vi "contract inside.vi"(10 "xmax":dbl[](array[numeric]), 11 "centroid":dbl[](array[numeric])) -> (3 "xc":dbl[](array[numeric]))   [LabVIEW 2015]
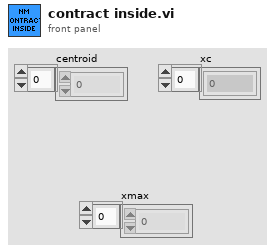
[diagram p1: front panel]
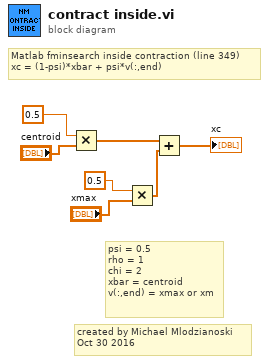
[diagram p0: block diagram]
diagram:
  # "Matlab fminsearch inside contraction (line 349)\nxc = (1-psi)*xbar + psi*v(:,end)"
  # "created by Michael Mlodzianoski\nOct 30 2016"
  # "psi = 0.5\nrho = 1\nchi = 2\nxbar = centroid\nv(:,end) = xmax or xm"
  n1 = Multiply(x=0.5, y="centroid") -> (x*y=w3:dbl[])
  n2 = Multiply(x=0.5, y="xmax") -> (x*y=w2:dbl[])
  n3 = Add(x=w3, y=w2) -> (x+y=→"xc":dbl[])
